vi "AFG3352X.ProcEvents.vi"(0 "i ref in":refnum<vi>, 5 "error in (no error)":errorcluster) -> (14 "i ref out":refnum<vi>, 19 "error out":errorcluster)   [LabVIEW 2014, in "AFG3352X.lvlib"]
doc: "This method is used to define the events the object will listen to. Add your own events here."
uses:
  AFG3352X.lvlib
  CSCore/BaseProcess/BaseProcess.event definition.ctl
  CSCore/CAEObj/CAEObj.event definition.ctl
  CSCore/BaseProcess/BaseProcess.descriptor string definition.ctl
  CSCore/BaseProcess/BaseProcess.lvlib
  CSCore/CAEObj/CAEObj.lvlib
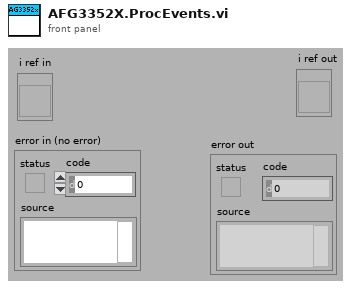
[diagram p1: front panel]
types:
  T1 = typedef "BaseProcess.lvlib/BaseProcess.event definition.ctl" = cluster{"CAEEvtDef":T2, "Data Descriptor":T3}
  T2 = typedef "CAEObj.lvlib/CAEObj.event definition.ctl" = cluster{"URL":string, "enable":bool, "ignoreResID":bool}
  T3 = typedef "BaseProcess.lvlib/BaseProcess.descriptor string definition.ctl" = string
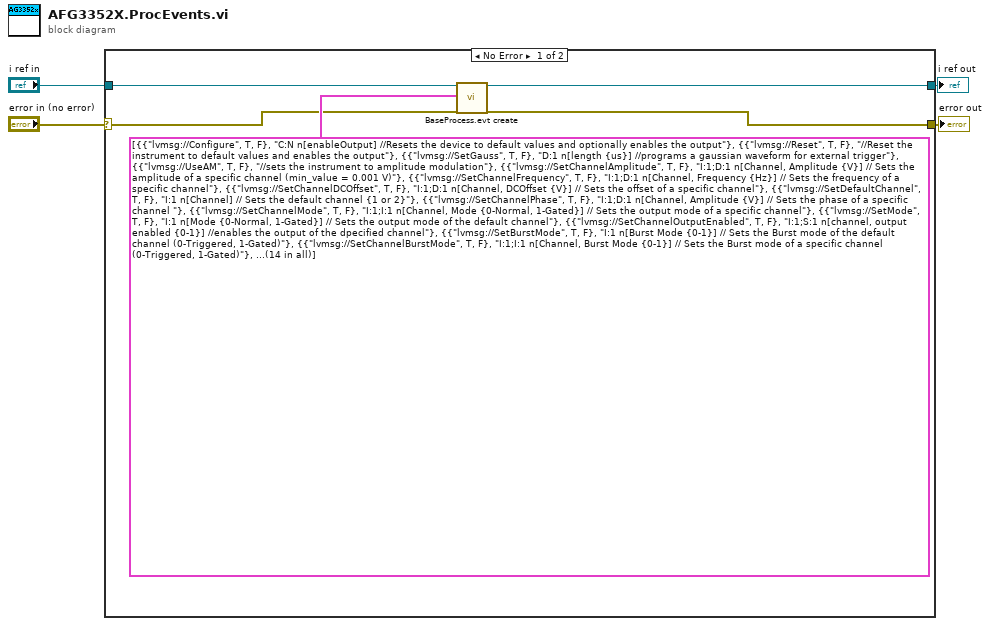
[diagram p0: block diagram]
diagram:
  n1 = case shown="No Error" "error in (no error)" {
    selector: "error in (no error)" -> [w5 w10]
    tunnel: "i ref in" -> [w9 w11]
    tunnel: [w8 w11] -> w3
    tunnel: [w7 w10] -> w2
    frame No Error {
      n2 = call "BaseProcess.evt create.vi"("i ref in"=w9, "newEvents"=T1[] [{"CAEEvtDef"={"URL"="lvmsg://Configure", "enable"=TRUE, "ignoreResID"=FALSE}, "Data Descriptor"="C:N n[enableOutput] //Resets the device to default values and optionally enables the output"}, {"CAEEvtDef"={"URL"="lvmsg://Reset", "enable"=TRUE, "ignoreResID"=FALSE}, "Data Descriptor"="//Reset the instrument to default values and enables the output"}, {"CAEEvtDef"={"URL"="lvmsg://SetGauss", "enable"=TRUE, "ignoreResID"=FALSE}, "Data Descriptor"="D:1 n[length {us}] //programs a gaussian waveform for external trigger"}, {"CAEEvtDef"={"URL"="lvmsg://UseAM", "enable"=TRUE, "ignoreResID"=FALSE}, "Data Descriptor"="//sets the instrument to amplitude modulation"}, {"CAEEvtDef"={"URL"="lvmsg://SetChannelAmplitude", "enable"=TRUE, "ignoreResID"=FALSE}, "Data Descriptor"="I:1;D:1 n[Channel, Amplitude {V}] // Sets the amplitude of a specific channel (min_value = 0.001 V)"}, {"CAEEvtDef"={"URL"="lvmsg://SetChannelFrequency", "enable"=TRUE, "ignoreResID"=FALSE}, "Data Descriptor"="I:1;D:1 n[Channel, Frequency {Hz}] // Sets the frequency of a specific channel"}, {"CAEEvtDef"={"URL"="lvmsg://SetChannelDCOffset", "enable"=TRUE, "ignoreResID"=FALSE}, "Data Descriptor"="I:1;D:1 n[Channel, DCOffset {V}] // Sets the offset of a specific channel"}, {"CAEEvtDef"={"URL"="lvmsg://SetDefaultChannel", "enable"=TRUE, "ignoreResID"=FALSE}, "Data Descriptor"="I:1 n[Channel] // Sets the default channel {1 or 2}"}, {"CAEEvtDef"={"URL"="lvmsg://SetChannelPhase", "enable"=TRUE, "ignoreResID"=FALSE}, "Data Descriptor"="I:1;D:1 n[Channel, Amplitude {V}] // Sets the phase of a specific channel "}, {"CAEEvtDef"={"URL"="lvmsg://SetChannelMode", "enable"=TRUE, "ignoreResID"=FALSE}, "Data Descriptor"="I:1;I:1 n[Channel, Mode {0-Normal, 1-Gated}] // Sets the output mode of a specific channel"}, {"CAEEvtDef"={"URL"="lvmsg://SetMode", "enable"=TRUE, "ignoreResID"=FALSE}, "Data Descriptor"="I:1 n[Mode {0-Normal, 1-Gated}] // Sets the output mode of the default channel"}, {"CAEEvtDef"={"URL"="lvmsg://SetChannelOutputEnabled", "enable"=TRUE, "ignoreResID"=FALSE}, "Data Descriptor"="I:1;S:1 n[channel, output enabled {0-1}] //enables the output of the dpecified channel"}, {"CAEEvtDef"={"URL"="lvmsg://SetBurstMode", "enable"=TRUE, "ignoreResID"=FALSE}, "Data Descriptor"="I:1 n[Burst Mode {0-1}] // Sets the Burst mode of the default channel (0-Triggered, 1-Gated)"}, {"CAEEvtDef"={"URL"="lvmsg://SetChannelBurstMode", "enable"=TRUE, "ignoreResID"=FALSE}, "Data Descriptor"="I:1;I:1 n[Channel, Burst Mode {0-1}] // Sets the Burst mode of a specific channel (0-Triggered, 1-Gated)"}] ("new events"), "error in (no error)"=w5) -> ("i ref out"=w8:refnum<vi>, "error out"=w7:errorcluster)  [unwired: 13 in, 2 out]
    }
    frame Error {
    }
  }
  "i ref out" <- w3
  "error out" <- w2
